vi "SetValueByHierarchicalPath.vi"(0 "VI Reference In":refnum<vi>, 2 "delimiter (>>)":string=">>", 5 "Control Path":string, 7 "Hierarchical Path":string, 11 "Error In":errorcluster) -> (4 "VI Reference Out":refnum<vi>, 15 "Error Out":errorcluster)   [LabVIEW 2016, in "Drona.lvlib" / "ControlValue.lvlib" / "StimulusTree.lvlib"]
doc: "Sets value(signaling) for the tree control whose item name is specified as a hierarchical path.\n\nHierarchical path represent their corresponding parents of an item from its origin. Use the delimiters '>>' between each hierarchy in the path.\n\nFor example to select the item 'Child3', give the hierarchical path as \"Parent1>>Child1>>Child2>>Child3\".\n\nThe input control name is given as a string , incase of path, use delimiters inbetween the path."
uses:
  StimulusTree.lvlib
  <vilib>/Utility/error.llb/Error Cluster From Error Code.vi
  <vilib>/ErrorRing/Error Ring.xnode
  Drona.lvlib
  Get/GetControlRef/GetControlRef.lvlib
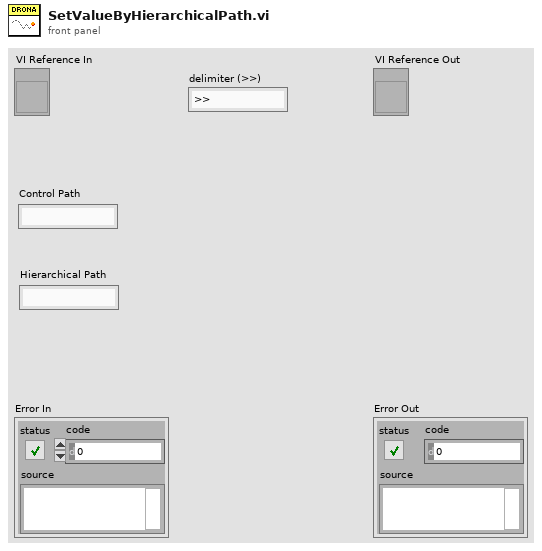
[diagram p1: front panel]
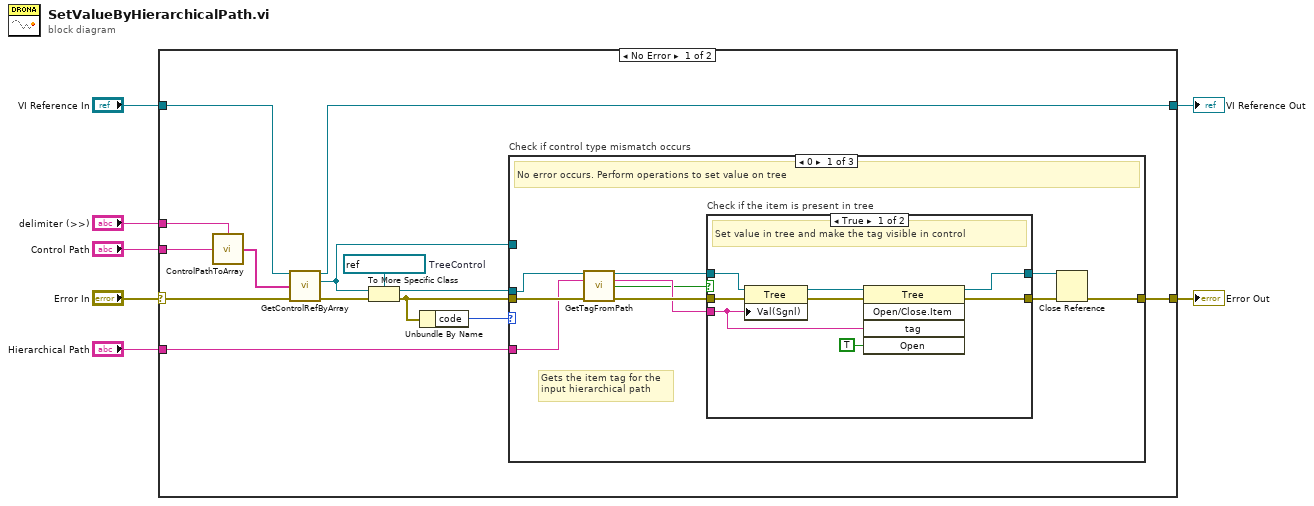
[diagram p0: block diagram]
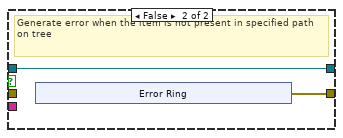
[diagram p2: hidden frame]
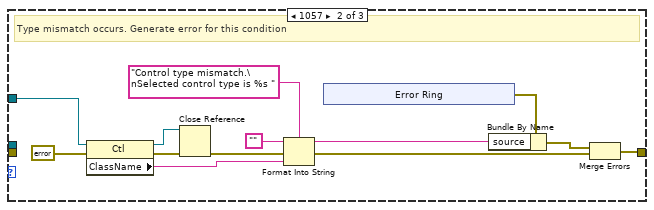
[diagram p3: hidden frame]
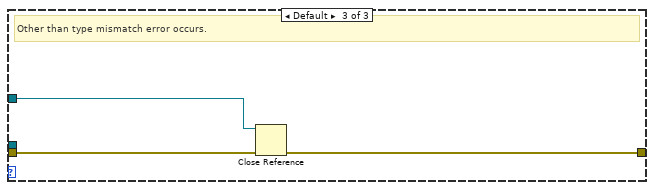
[diagram p4: hidden frame]
diagram:
  n1 = case shown="No Error" "Error In" {
    selector: "Error In" -> [w18 w69]
    tunnel: [w8 w69] -> w6
    tunnel: "VI Reference In" -> [w17 w68]
    tunnel: "Control Path" -> [w20 _]
    tunnel: [w14 w68] -> w3
    tunnel: "delimiter (>>)" -> [w19 _]
    tunnel: "Hierarchical Path" -> [w9 _]
    frame No Error {
      w21 = refnum<vi> refnum  # TreeControl
      n2 = call "ControlPathToArray.vi"("Control Name"=w20, "delimiter (>>)"=w19) -> ("Control Path"=w16:string[])
      n3 = call "GetControlRefByArray.vi"("VI Reference In"=w17, "Control Path"=w16, "error In"=w18) -> ("VI Reference Out"=w14:refnum<vi>, "Ctl Refnum"=w13:refnum<vi>, "error out"=w15:errorcluster)  [unwired: 10 in]
      n4 = To More Specific Class(target class=w21, reference=w13, error in=w15) -> (specific class reference=w12:refnum<vi>, error out=w11:errorcluster)
      n5 = Unbundle By Name(w11) -> ("code"=w10:i32)
      n6 = case "Check if control type mismatch occurs" shown="0" w10 {
        tunnel: [w31 w49 w66] -> w8
        tunnel: w12 -> [w26 _ _]
        tunnel: w13 -> [_ w59 w65]
        tunnel: w11 -> [w28 _ w67]
        tunnel: w9 -> [w25 _ _]
        frame 0 {
          # "Gets the item tag for the \ninput hierarchical path"
          # "No error occurs. Perform operations to set value on tree"
          n7 = call "GetTagFromPath.vi"("Tree Ref In"=w26, "Hierarchical Path"=w25, "Error In"=w28) -> ("Tree Ref Out"=w24:refnum<vi>, "Item Tag"=w23:string, "Item Found?"=w22:bool, "Error Out"=w27:errorcluster)  [unwired: 9 in]
          n8 = case "Check if the item is present in tree" shown="True" w22 {
            tunnel: [w38 w41] -> w30
            tunnel: [w35 w40] -> w29
            tunnel: w24 -> [w34 w40]
            tunnel: w23 -> [w32 _]
            tunnel: w27 -> [w33 _]
            frame True {
              # "Set value in tree and make the tag visible in control"
              n9 = property class="Tree"(reference=w34, error in=w33, "Val(Sgnl)"=w32) -> (reference out=w37:refnum<vi>, error out=w39:errorcluster)
              n10 = invoke class="Tree" method="Open/Close.Item"(reference=w37, error in=w39, "tag"=w32, "Open"=TRUE ("Open?")) -> (reference out=w35:refnum<vi>, error out=w38:errorcluster)  [unwired: 1 in, 3 out]
            }
            frame False {
              # "Generate error when the item is not present in specified path on tree"
              n11 = xnode "Error Ring"() -> ("error out"=w41:errorcluster)
            }
          }
          n12 = Close Reference(reference=w29, error in (no error)=w30) -> (error out=w31:errorcluster)
        }
        frame 1057 {
          # "Type mismatch occurs. Generate error for this condition"
          n13 = property class="Ctl"(reference=w59, error in=errorcluster {"status"=FALSE, "code"=0, "source"=""} ("error out")) -> (reference out=w47:refnum<vi>, error out=w58:errorcluster, "ClassName"=w55:string)
          n14 = Close Reference(reference=w47, error in (no error)=w58) -> (error out=w48:errorcluster)
          n15 = Format Into String(format string="Control type mismatch.\nSelected control type is %s ", initial string="", error in=w48, w55) -> (resulting string=w52:string, error out=w50:errorcluster)
          n16 = xnode "Error Ring"() -> ("error out"=w53:errorcluster)
          n17 = Bundle By Name(cluster=w53, "source"=w52) -> (w51:errorcluster)
          n18 = Merge Errors(w51, w50) -> (w49:errorcluster)
        }
        frame Default {
          # "Other than type mismatch error occurs."
          n19 = Close Reference(reference=w65, error in (no error)=w67) -> (error out=w66:errorcluster)
        }
      }
    }
    frame Error {
    }
  }
  "Error Out" <- w6
  "VI Reference Out" <- w3
